vi "Install Support_Post-Uninstall Custom Action.vi"(10 "Variant":variant) -> (0 "error out":errorcluster)   [LabVIEW 2021]
uses:
  <vilib>/zip/NI_Unzip.lvlib
  <vilib>/Utility/config.llb/NI_LVConfig.lvlib
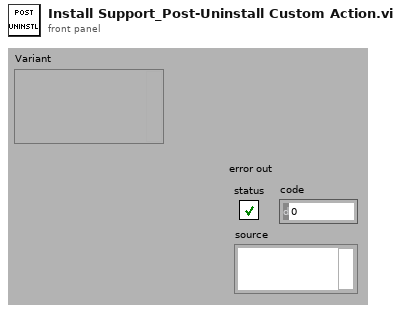
[diagram p1: front panel]
types:
  T1 = typedef "NI_LVConfig.lvlib/Config Data RefNum.ctl" = refnum<k1>
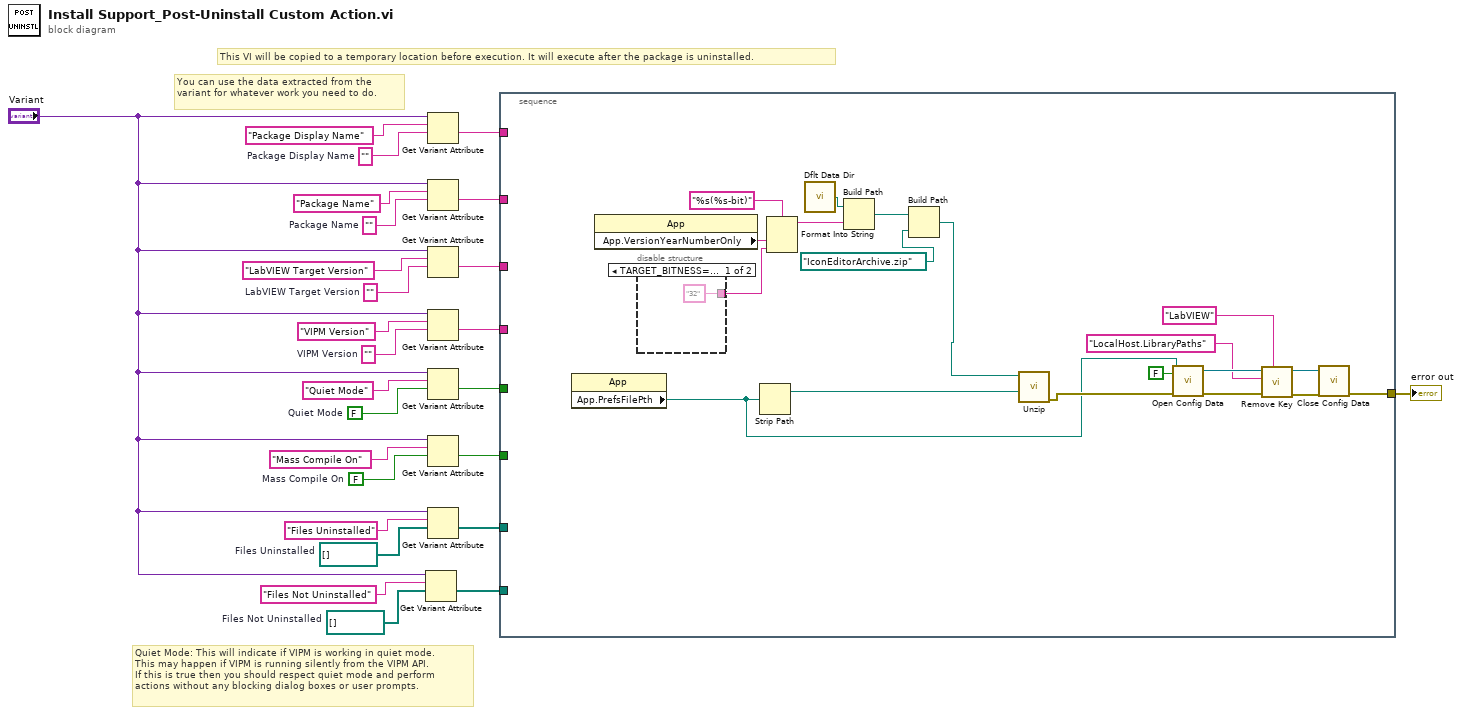
[diagram p0: block diagram]
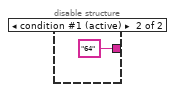
[diagram p2: hidden frame]
diagram:
  w2 = path[] []  # Files Not Uninstalled
  w3 = path[] []  # Files Uninstalled
  w9 = FALSE  # Mass Compile On
  w10 = ""  # Package Display Name
  w17 = FALSE  # Quiet Mode
  w20 = ""  # VIPM Version
  w22 = ""  # LabVIEW Target Version
  w24 = ""  # Package Name
  # "You can use the data extracted from the variant for whatever work you need to do."
  # "Quiet Mode: This will indicate if VIPM is working in quiet mode.\nThis may happen if VIPM is running silently from the VIPM API.\nIf this is true then you should respect quiet mode and perform\nactions without any blocking dialog boxes or user prompts."
  # "This VI will be copied to a temporary location before execution. It will execute after the package is uninstalled."
  n1 = Get Variant Attribute(Variant="Variant", name="Files Not Uninstalled", default value (empty Variant)=w2) -> (value=w7:path[])  [unwired: 1 in, 3 out]
  n2 = Get Variant Attribute(Variant="Variant", name="Package Display Name", default value (empty Variant)=w10) -> (value=w16:string)  [unwired: 1 in, 3 out]
  n3 = Get Variant Attribute(Variant="Variant", name="Package Name", default value (empty Variant)=w24) -> (value=w15:string)  [unwired: 1 in, 3 out]
  n4 = Get Variant Attribute(Variant="Variant", name="LabVIEW Target Version", default value (empty Variant)=w22) -> (value=w14:string)  [unwired: 1 in, 3 out]
  n5 = Get Variant Attribute(Variant="Variant", name="VIPM Version", default value (empty Variant)=w20) -> (value=w13:string)  [unwired: 1 in, 3 out]
  n6 = Get Variant Attribute(Variant="Variant", name="Quiet Mode", default value (empty Variant)=w17) -> (value=w12:bool)  [unwired: 1 in, 3 out]
  n7 = Get Variant Attribute(Variant="Variant", name="Mass Compile On", default value (empty Variant)=w9) -> (value=w11:bool)  [unwired: 1 in, 3 out]
  n8 = Get Variant Attribute(Variant="Variant", name="Files Uninstalled", default value (empty Variant)=w3) -> (value=w6:path[])  [unwired: 1 in, 3 out]
  n9 = stacked-sequence {
    tunnel: w16 -> [_]
    tunnel: w15 -> [_]
    tunnel: w14 -> [_]
    tunnel: w13 -> [_]
    tunnel: w12 -> [_]
    tunnel: w11 -> [_]
    tunnel: w6 -> [_]
    tunnel: w7 -> [_]
    tunnel: [w31] -> w1
    frame #0 {
      n10 = property class="App"() -> ("App.PrefsFilePth"=w27:path)  [unwired: 2 in, 2 out]
      n11 = property class="App"() -> ("App.VersionYearNumberOnly"=w38:string)  [unwired: 2 in, 2 out]
      n12 = disable-structure shown="TARGET_BITNESS==32" {
        disable-tunnel: ["32" "64"] -> w39
        frame condition #0 {
        }
        frame condition #1 (active) {
        }
      }
      n13 = Strip Path(path=w27) -> (stripped path=w29:path)  [unwired: 1 out]
      n14 = Format Into String(format string="%s(%s-bit)", w38, w39) -> (resulting string=w40:string)  [unwired: 2 in, 1 out]
      n15 = call <vilib>:"Dflt Data Dir.vi"() -> ("App:Default Data Directory"=w44:path)
      n16 = Build Path(base path=w44, name or relative path=w40) -> (appended path=w43:path)
      n17 = Build Path(base path=w43, name or relative path=path "IconEditorArchive.zip") -> (appended path=w41:path)
      n18 = call <vilib>:"Unzip.vi"("Target directory (same as Zip file if empty)"=w29, "Zip file"=w41) -> ("error out"=w28:errorcluster)  [unwired: 7 in, 2 out]
      n19 = call <vilib>:"Open Config Data.vi"("error in (no error)"=w28, "create file if necessary (T)"=FALSE, "configuration file path"=w27) -> ("error out"=w37:errorcluster, "refnum"=w36:T1)  [unwired: 6 in, 1 out]
      n20 = call <vilib>:"Remove Key.vi"("section"="LabVIEW", "error in (no error)"=w37, "key"="LocalHost.LibraryPaths", "refnum"=w36) -> ("error out"=w33:errorcluster, "refnum out"=w32:T1)  [unwired: 5 in, 1 out]
      n21 = call <vilib>:"Close Config Data.vi"("error in (no error)"=w33, "refnum"=w32) -> ("error out"=w31:errorcluster)  [unwired: 8 in, 1 out]
    }
  }
  "error out" <- w1
